vi "set_global_variables.vi"(4 "State":i16, 5 "Time":dbl format="%.2f", 6 "Sensor Values":dbl[](array[numeric]), 7 "Set Points":dbl[](array[numeric])) -> (0 "required data":T1={"Set Point names"=["height_ff(m)", "C_coag_stock(g/L)", "flocculation_time(min)", "clarification_time(min)", "data_interval(min)", "kpf", "kc", "q"], "required number of setpoints"=8, "required number of sensors"=0, "Sensor names"=[""]}, 3 "output value":dbl)   [LabVIEW 2019]
uses:
  Global Plantita Parameters.vi
panel:
  # "Enter the correct information for this control code in the required data structure below. Then make the current value default by right clicking on the border of the data structure. Select \"data operations\" and then select \"make current value default\". These values will be displayed by process controller."
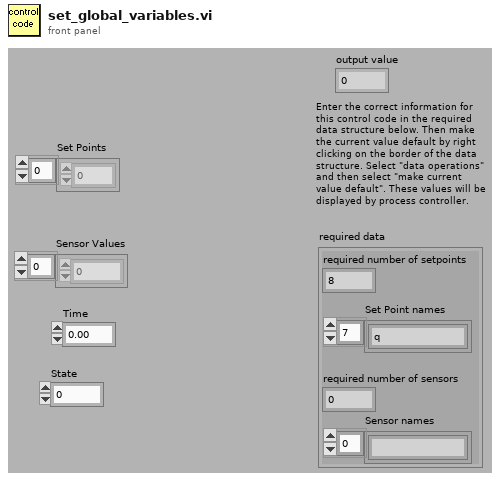
[diagram p1: front panel]
types:
  T1 = cluster{"Set Point names":string[], "required number of setpoints":u8, "required number of sensors":u8, "Sensor names":string[]}
  T2 = cluster{"height_ff (m)":dbl, "C_coag_stock (g/L)":dbl, "flocculation_time(min)":dbl, "clarification_time(min)":dbl, "data_interval (min)":dbl, "kpf":dbl, "kc":dbl, "q":dbl}
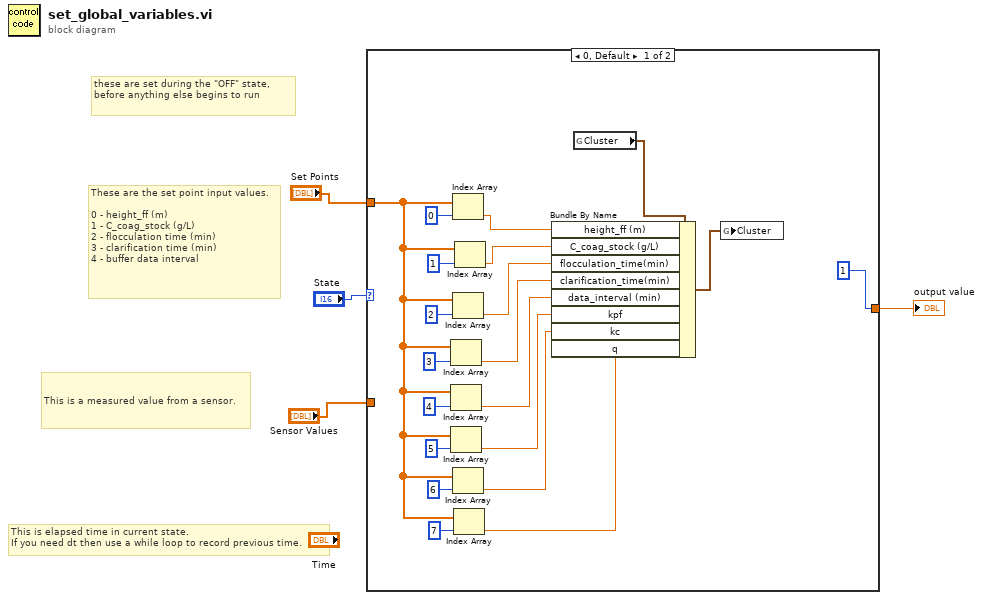
[diagram p0: block diagram]
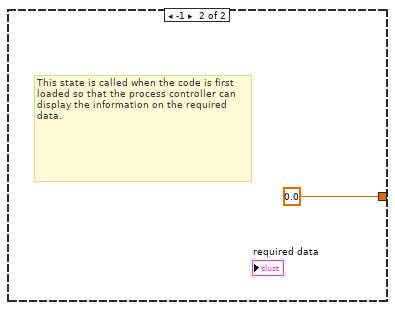
[diagram p2: hidden frame]
diagram:
  # "these are set during the \"OFF\" state, before anything else begins to run"
  # "These are the set point input values.\n\n0 - height_ff (m)\n1 - C_coag_stock (g/L)\n2 - flocculation time (min)\n3 - clarification time (min)\n4 - buffer data interval"
  # "This is a measured value from a sensor."
  # "This is elapsed time in current state.\nIf you need dt then use a while loop to record previous time."
  n1 = case shown="0, Default" "State" {
    tunnel: [1 0.0 ("fraction on")] -> w1
    tunnel: "Set Points" -> [w7 _]
    tunnel: "Sensor Values" -> [_ _]
    frame 0, Default {
      n2 = Index Array(array=w7, index=3) -> (element=w12:dbl)
      n3 = Index Array(array=w7, index=4) -> (element=w13:dbl)
      n4 = Index Array(array=w7, index=5) -> (element=w10:dbl)
      n5 = Index Array(array=w7, index=0) -> (element=w19:dbl)
      n6 = Index Array(array=w7, index=2) -> (element=w16:dbl)
      n7 = Index Array(array=w7, index=6) -> (element=w6:dbl)
      n8 = Index Array(array=w7, index=7) -> (element=w5:dbl)
      n9 = Index Array(array=w7, index=1) -> (element=w18:dbl)
      n10 = global read "Global Plantita Parameters.vi" "Cluster"() -> (w20:T2)
      n11 = Bundle By Name(cluster=w20, "height_ff (m)"=w19, "C_coag_stock (g/L)"=w18, "flocculation_time(min)"=w16, "clarification_time(min)"=w12, "data_interval (min)"=w13, "kpf"=w10, "kc"=w6, "q"=w5) -> (w21:T2)
      n12 = global write "Global Plantita Parameters.vi" "Cluster"(w21) -> ()
    }
    frame -1 {
      # "This state is called when the code is first loaded so that the process controller can display the information on the required data."
    }
  }
  "output value" <- w1
